vi "freqSet.vi"(7 "ms to wait (1000)":u32=1000, 8 "error in (no error)":errorcluster, 9 "laser":u16(ring) items=["blue", "green", "red", "ir"], 10 "Freq, Hz (1370)":i32=1370, 11 "Teensy Port":refnum<visa-resource-name>) -> (0 "error out":errorcluster, 3 "VISA Refnum out":refnum<visa-resource-name>)   [LabVIEW 2011]
panel:
  out "resulting string":string
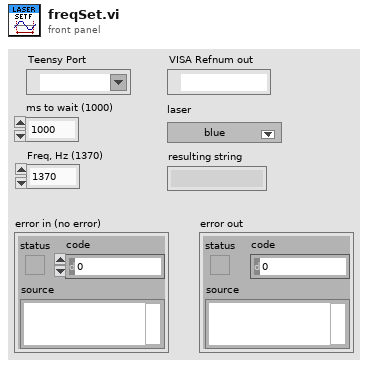
[diagram p1: front panel]
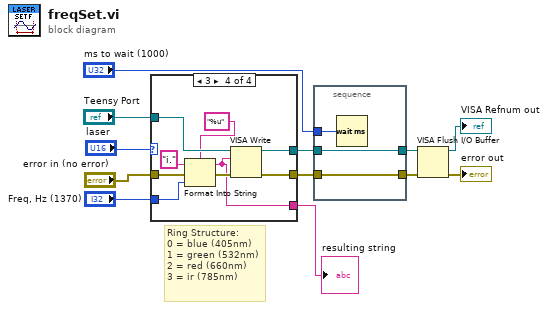
[diagram p0: block diagram]
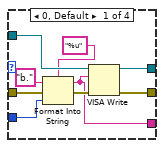
[diagram p2: hidden frame]
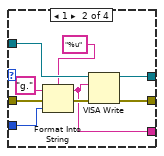
[diagram p3: hidden frame]
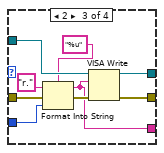
[diagram p4: hidden frame]
diagram:
  # "Ring Structure:\n0 = blue (405nm)\n1 = green (532nm)\n2 = red (660nm)\n3 = ir (785nm)"
  n1 = case shown="3" "laser" {
    tunnel: [w21 w30 w39 w48] -> w2
    tunnel: [w20 w29 w38 w47] -> w3
    tunnel: "error in (no error)" -> [w18 w27 w36 w45]
    tunnel: "Teensy Port" -> [w17 w26 w35 w44]
    tunnel: "Freq, Hz (1370)" -> [w16 w25 w34 w43]
    tunnel: [w13 w22 w31 w40] -> w1
    frame 0, Default {
      n2 = Format Into String(format string="%u", initial string="b.", error in=w18, w16) -> (resulting string=w13:string, error out=w19:errorcluster)
      n3 = VISA Write(VISA resource name=w17, write buffer=w13, error in (no error)=w19) -> (VISA resource name out=w21:refnum<visa-resource-name>, error out=w20:errorcluster)  [unwired: 1 out]
    }
    frame 1 {
      n4 = Format Into String(format string="%u", initial string="g.", error in=w27, w25) -> (resulting string=w22:string, error out=w28:errorcluster)
      n5 = VISA Write(VISA resource name=w26, write buffer=w22, error in (no error)=w28) -> (VISA resource name out=w30:refnum<visa-resource-name>, error out=w29:errorcluster)  [unwired: 1 out]
    }
    frame 2 {
      n6 = Format Into String(format string="%u", initial string="r.", error in=w36, w34) -> (resulting string=w31:string, error out=w37:errorcluster)
      n7 = VISA Write(VISA resource name=w35, write buffer=w31, error in (no error)=w37) -> (VISA resource name out=w39:refnum<visa-resource-name>, error out=w38:errorcluster)  [unwired: 1 out]
    }
    frame 3 {
      n8 = Format Into String(format string="%u", initial string="i.", error in=w45, w43) -> (resulting string=w40:string, error out=w46:errorcluster)
      n9 = VISA Write(VISA resource name=w44, write buffer=w40, error in (no error)=w46) -> (VISA resource name out=w48:refnum<visa-resource-name>, error out=w47:errorcluster)  [unwired: 1 out]
    }
  }
  "resulting string" <- w1
  n10 = stacked-sequence {
    tunnel: w3 -> [w50]
    tunnel: w2 -> [w51]
    tunnel: [w51] -> w6
    tunnel: [w50] -> w7
    tunnel: "ms to wait (1000)" -> [w49]
    frame #0 {
      n11 = Wait (ms)(milliseconds to wait=w49) -> ()  [unwired: 1 out]
    }
  }
  n12 = VISA Flush I/O Buffer(VISA resource name=w6, error in (no error)=w7) -> (VISA resource name out=→"VISA Refnum out":refnum<visa-resource-name>, error out=→"error out":errorcluster)  [unwired: 1 in]
